vi "Access Data.vi"(8 "error in (no error)":errorcluster, 10 "Index":i32, 11 "2D U16 DVR Array in":refnum<class "2D U16 DVR Array.lvclass">) -> (0 "error out":errorcluster, 2 "Array Out":u16[][](array[numeric]), 3 "2D U16 DVR Array out":refnum<class "2D U16 DVR Array.lvclass">)   [LabVIEW 2024, in "2D U16 DVR Array.lvclass"]
uses:
  2D U16 DVR Array.lvclass
  2D U16 DVR Array.lvclass/2D U16 DVR Array.ctl
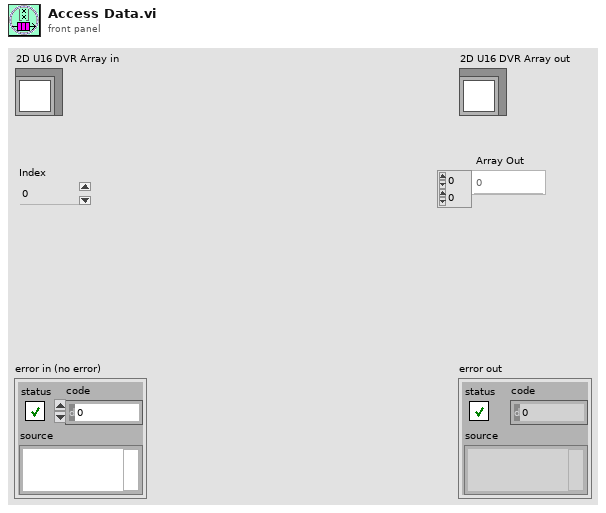
[diagram p1: front panel]
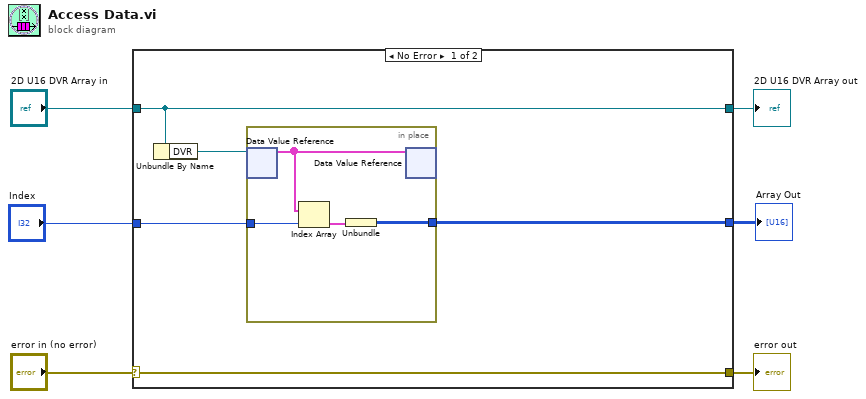
[diagram p0: block diagram]
diagram:
  n1 = case shown="No Error" "error in (no error)" {
    selector: "error in (no error)" -> [w11 w17]
    tunnel: [w11 w17] -> w5
    tunnel: [w10 w16] -> w3
    tunnel: "2D U16 DVR Array in" -> [w10 w16]
    tunnel: "Index" -> [w8 _]
    tunnel: [w7 _] -> w1
    frame No Error {
      n2 = Unbundle By Name(w10) -> ("DVR"=w9:refnum<data-value>)
      n3 = in-place {
        in-place-border: w8 -> [w14]
        in-place-border: [w12] -> w7
        n4 = in-place-dvr #1(w9) -> (w15:cluster{u16[][]}[])  [unwired: 1 out]
        n5 = Index Array(array=w15, index=w14) -> (element=w13:cluster{u16[][]})
        n6 = Unbundle(w13) -> (w12:u16[][])
        n7 = in-place-dvr #1(w15) -> ()  [unwired: 2 out]
      }
    }
    frame Error {
    }
  }
  "error out" <- w5
  "2D U16 DVR Array out" <- w3
  "Array Out" <- w1
